vi "Material-VacuumControl.vi"(8 "error in (no error)":errorcluster, 11 "Vacuum On/Off":bool) -> (0 "error out":errorcluster)   [LabVIEW 2013, in "Material-RunTest.lvclass"]
uses:
  Material-RunTest.lvclass
  <vilib>/DAQmx/write.llb/DAQmx Write (Digital 1D Bool NChan 1Samp 1Line).vi
  <vilib>/DAQmx/write.llb/DAQmx Write (Digital Bool 1Line 1Point).vi
  <vilib>/DAQmx/create/channels.llb/DAQmx Create Channel (DO-Digital Output).vi
  <vilib>/DAQmx/miscellaneous.llb/DAQmx Fill In Error Info.vi
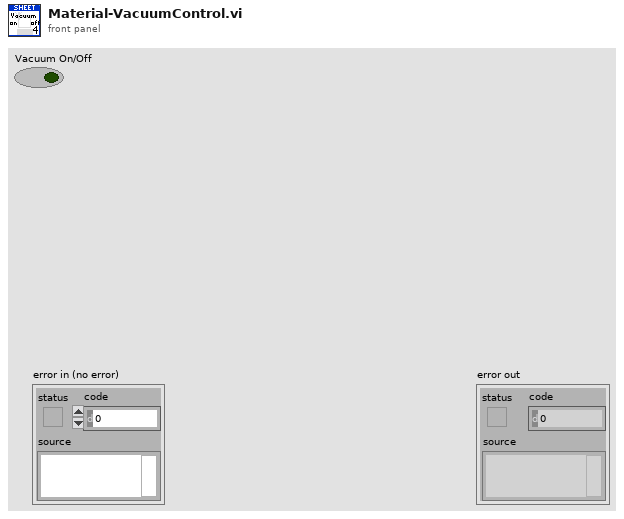
[diagram p1: front panel]
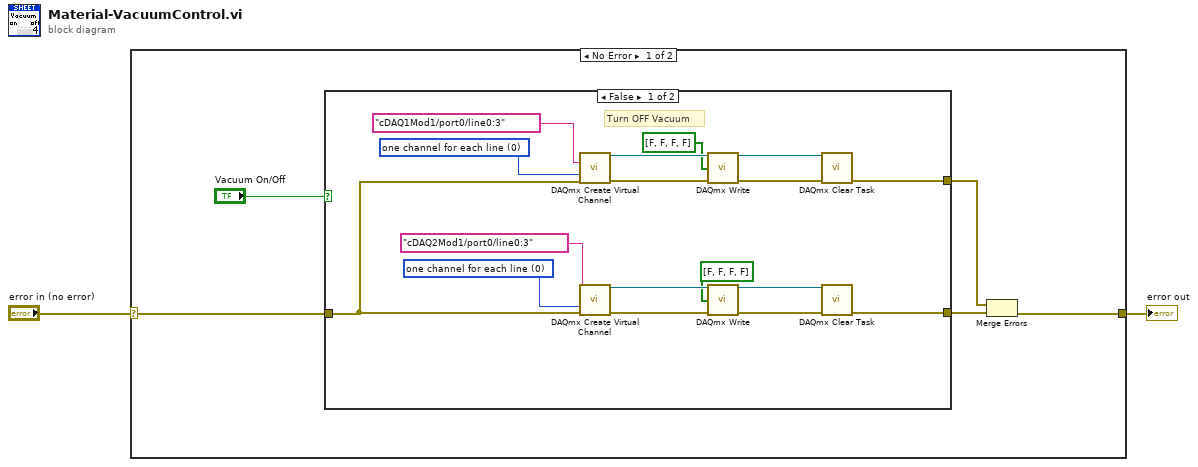
[diagram p0: block diagram]
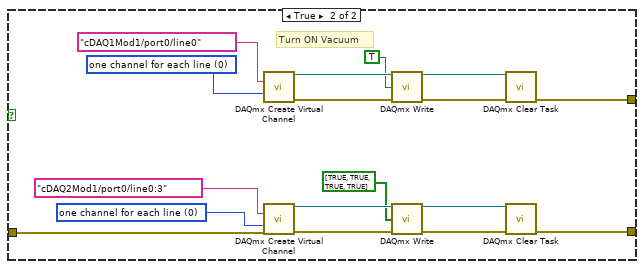
[diagram p2: hidden frame]
diagram:
  n1 = case shown="No Error" "error in (no error)" {
    selector: "error in (no error)" -> [w7 w42]
    tunnel: [w4 w42] -> w1
    frame No Error {
      n2 = case shown="False" "Vacuum On/Off" {
        tunnel: w7 -> [w10 w25]
        tunnel: [w9 w27] -> w6
        tunnel: [w8 w26] -> w5
        frame False {
          w13 = 0 items=["one channel for each line", "one channel for all lines"] ("line grouping")
          w23 = 0 items=["one channel for each line", "one channel for all lines"] ("line grouping")
          # "Turn OFF Vacuum"
          n3 = call-poly <vilib>:"DAQmx Create Virtual Channel.vi"("lines"=tag "cDAQ1Mod1/port0/line0:3", "line grouping"=w23, "error in"=w10) -> ("task out"=w22:refnum<k21>, "error out"=w21:errorcluster)  [unwired: 11 in]
          n4 = call-poly <vilib>:"DAQmx Create Virtual Channel.vi"("lines"=tag "cDAQ2Mod1/port0/line0:3", "line grouping"=w13, "error in"=w10) -> ("task out"=w14:refnum<k21>, "error out"=w15:errorcluster)  [unwired: 11 in]
          n5 = call-poly <vilib>:"DAQmx Write.vi"("task/channels in"=w22, "data"=bool[] [FALSE, FALSE, FALSE, FALSE] ("data 4"), "error in"=w21) -> ("task out"=w20:refnum<k21>, "error out"=w19:errorcluster)  [unwired: 10 in, 1 out]
          n6 = call-poly <vilib>:"DAQmx Write.vi"("task/channels in"=w14, "data"=bool[] [FALSE, FALSE, FALSE, FALSE] ("data 3"), "error in"=w15) -> ("task out"=w16:refnum<k21>, "error out"=w17:errorcluster)  [unwired: 10 in, 1 out]
          n7 = call <vilib>:"DAQmx Clear Task.vi"("task in"=w20, "error in"=w19) -> ("error out"=w9:errorcluster)  [unwired: 13 in]
          n8 = call <vilib>:"DAQmx Clear Task.vi"("task in"=w16, "error in"=w17) -> ("error out"=w8:errorcluster)  [unwired: 13 in]
        }
        frame True {
          w32 = 0 items=["one channel for each line", "one channel for all lines"] ("line grouping")
          w41 = 0 items=["one channel for each line", "one channel for all lines"] ("line grouping")
          # "Turn ON Vacuum"
          n9 = call-poly <vilib>:"DAQmx Create Virtual Channel.vi"("lines"=tag "cDAQ1Mod1/port0/line0", "line grouping"=w41) -> ("task out"=w40:refnum<k21>, "error out"=w39:errorcluster)  [unwired: 12 in]
          n10 = call-poly <vilib>:"DAQmx Create Virtual Channel.vi"("lines"=tag "cDAQ2Mod1/port0/line0:3", "line grouping"=w32, "error in"=w25) -> ("task out"=w33:refnum<k21>, "error out"=w34:errorcluster)  [unwired: 11 in]
          n11 = call-poly <vilib>:"DAQmx Write.vi"("task/channels in"=w40, "data"=TRUE ("Boolean"), "error in"=w39) -> ("task out"=w38:refnum<k21>, "error out"=w37:errorcluster)  [unwired: 10 in, 1 out]
          n12 = call-poly <vilib>:"DAQmx Write.vi"("task/channels in"=w33, "data"=bool[] [TRUE, TRUE, TRUE, TRUE] ("data 2"), "error in"=w34) -> ("task out"=w35:refnum<k21>, "error out"=w36:errorcluster)  [unwired: 10 in, 1 out]
          n13 = call <vilib>:"DAQmx Clear Task.vi"("task in"=w38, "error in"=w37) -> ("error out"=w27:errorcluster)  [unwired: 13 in]
          n14 = call <vilib>:"DAQmx Clear Task.vi"("task in"=w35, "error in"=w36) -> ("error out"=w26:errorcluster)  [unwired: 13 in]
        }
      }
      n15 = Merge Errors(w6, w5) -> (w4:errorcluster)
    }
    frame Error {
    }
  }
  "error out" <- w1
